vi "Example1.vi"   [LabVIEW 2018]
uses:
  src/MPU.lvclass
  <vilib>/rvi/DataTransferAndStorage/Container/Common/niFpgaContainerGetUniqueNameForEmu.vi
  <vilib>/rvi/DataTransferAndStorage/Container/Common/niFpgaContainerSetEmuInfo.vi
  <vilib>/rvi/eio/common/nirviEmuReportErrorAndStop.vi
  <vilib>/rvi/LocalResourceManager/LocalResourceManager.xnode
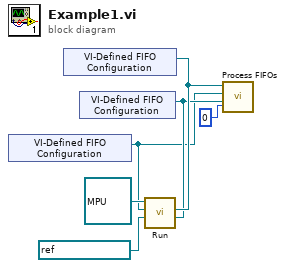
[diagram p0: block diagram]
diagram:
  n1 = xnode "VI-Defined FIFO Configuration"() -> ("FIFO Out"=w1:refnum<k21>)
  n2 = xnode "VI-Defined FIFO Configuration"() -> ("FIFO Out"=w4:refnum<k21>)
  n3 = xnode "VI-Defined FIFO Configuration"() -> ("FIFO Out"=w3:refnum<k21>)
  n4 = call-dynamic "Run.vi"("DebugOut"=w3, "Telemetry"=w4, "Port"=refnum<k21> "Mod1\\Port1", "Command FIFO"=w1, "MPU in"=refnum<class "MPU.lvclass"> refnum ("Modbus_Processing_Unit.lvlib:MPU.lvclass")) -> ()  [unwired: 4 in, 2 out]
  n5 = call "Process FIFOs.vi"("Timeout"=0, "FIFO Out 2"=w3, "FIFO Out"=w1, "Refnum in"=w4) -> ()  [unwired: 7 in, 1 out]
